vi "Test format.vi"() -> ()   [LabVIEW 2015]
uses:
  <vilib>/Utility/tdmsutil.llb/TDMS Create Scaling Information (Linear).vi
panel:
  out "scale array":dbl[][](array[numeric])
  in  "channel name(s) in (Untitled)":string[](array[string])
  out "output array":i32[][](array[numeric])
  in  "Array - Numeric":i32[](array[numeric])
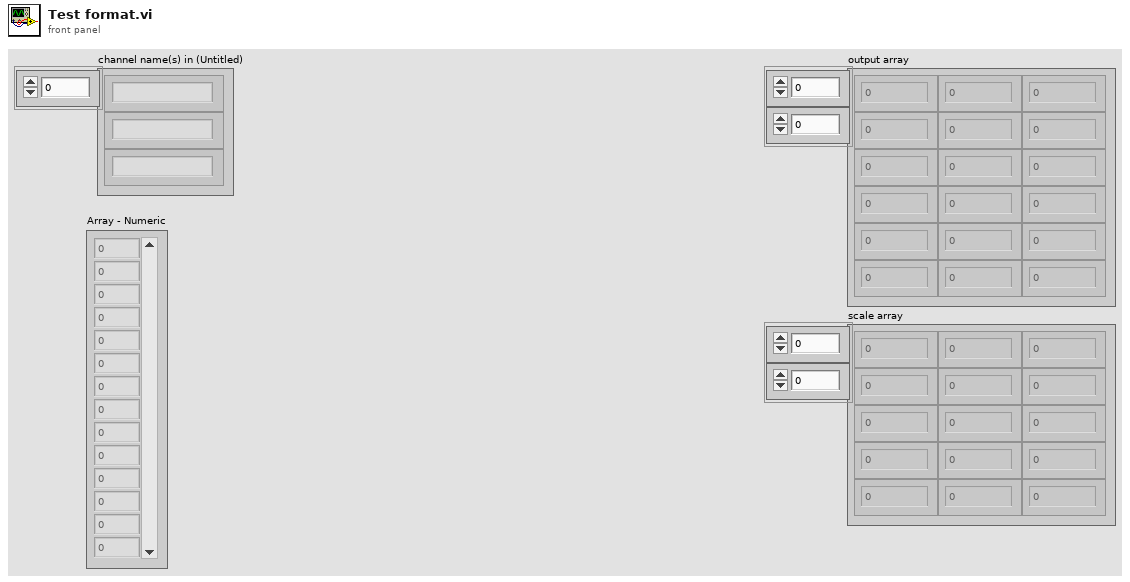
[diagram p1: front panel]
types:
  T1 = enum16{"open", "open or create", "create or replace", "create", "open (read-only)"}
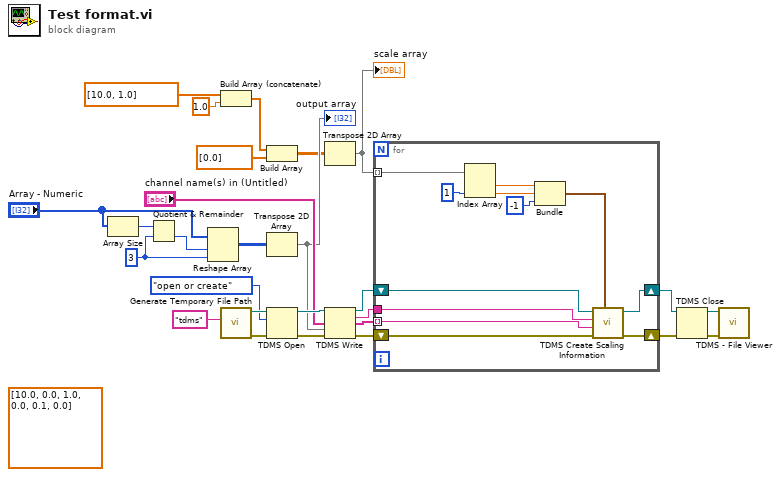
[diagram p0: block diagram]
diagram:
  (unwired) dbl[][] [[10.0, 0.0], [1.0, 0.0], [0.1, 0.0]]
  w7 = 3 ("dimension size")
  n1 = Array Size(array="Array - Numeric") -> (size(s)=w26:i32)
  n2 = Quotient & Remainder(x=w26, y=w7) -> (floor(x/y)=w8:i32)  [unwired: 1 out]
  n3 = Reshape Array("Array - Numeric", w8, w7) -> (w22:i32[][])
  n4 = Build Array (concatenate)(dbl[] [10.0, 1.0], 1.0) -> (w4:dbl[])
  n5 = call <vilib>:"Generate Temporary File Path.vi"("Temporary File Extension (tmp)"="tdms") -> ("error out"=w10:errorcluster, "Unique Temporary File Path"=w24:path)  [unwired: 9 in]
  n6 = Build Array(w4, dbl[] [0.0]) -> (w2:dbl[][])
  n7 = Transpose 2D Array(2D array=w22) -> (transposed array=w9:i32[][])
  "output array" <- w9
  n8 = TDMS Open(8:w10, 10:T1."open or create" ("operation (0:open)"), 11:w24) -> (0:w20:errorcluster, 3:w23:refnum<k34>)  [unwired: 4 in]
  n9 = Transpose 2D Array(2D array=w2) -> (transposed array=w1:dbl[][])
  "scale array" <- w1
  n10 = TDMS Write(0:w23, 7:"channel name(s) in (Untitled)", 9:w9, 11:w20) -> (4:w19:refnum<k34>, 6:w18:string, 8:w17:string[], 15:w16:errorcluster)  [unwired: 2 in]
  n11 = for {
    tunnel: w18 -> [w38]
    tunnel: w17 -> [w37] mode=indexing
    shift-right: [w35] -> w15
    shift-left: w16 -> [w36]
    shift-right: [w34] -> w14
    shift-left: w19 -> [w39]
    tunnel: w1 -> [w32] mode=indexing
    n12 = Index Array(array=w32, index #2=1 ("index")) -> (element #1=w30:dbl, element #2=w29:dbl)  [unwired: 1 in]
    n13 = Bundle(w30, w29, -1) -> (w28:cluster{dbl, dbl, i32})  [unwired: 1 in]
    n14 = call-poly <vilib>:"TDMS Create Scaling Information.vi"("linear scale"=w28, "error in (no error)"=w36, "channel name"=w37, "group name"=w38, "tdms file"=w39) -> ("error out"=w35:errorcluster, "tdms file out"=w34:refnum<k34>)  [unwired: 2 in, 3 out]
  }
  n15 = TDMS Close(8:w15, 11:w14) -> (0:w13:errorcluster, 3:w12:path)
  n16 = call <vilib>:"TDMS - File Viewer.vi"("error in (no error)"=w13, "file path"=w12) -> ()  [unwired: 4 in, 2 out]
